vi "get_image_type.vi"(8 "error in (no error)":errorcluster, 11 "Image.lvclass in":refnum<class "Image.lvclass">) -> (0 "error out":errorcluster, 2 "Image Type":T1 items=["Grayscale (U8)", "Grayscale (I16)", "Grayscale (SGL)", "Complex (CSG)", "RGB (U32)", "HSL (U32)", "RGB (U64)", "Grayscale (U16)"], 3 "Image.lvclass out":refnum<class "Image.lvclass">, 4 "bytes per pixel":i32)   [LabVIEW 2010, in "Image.lvclass"]
uses:
  Image.lvclass
  Image.lvclass/Image.ctl
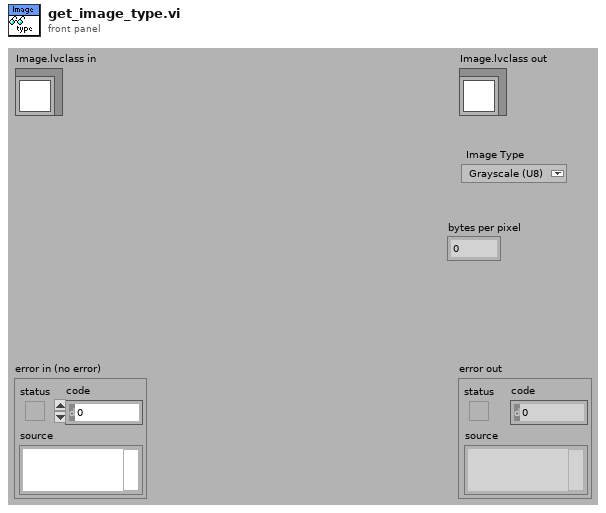
[diagram p1: front panel]
types:
  T1 = typedef "Image Type" = u32
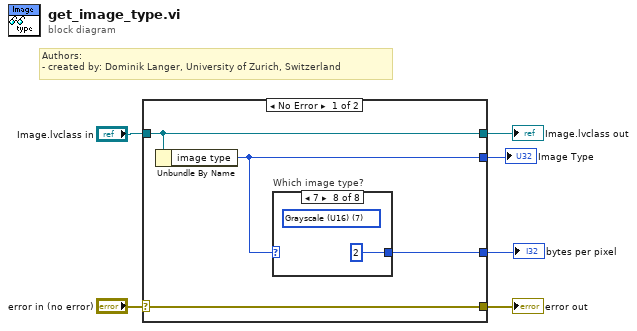
[diagram p0: block diagram]
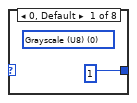
[diagram p2: hidden frame]
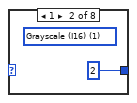
[diagram p3: hidden frame]
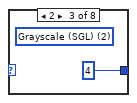
[diagram p4: hidden frame]
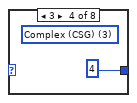
[diagram p5: hidden frame]
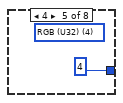
[diagram p6: hidden frame]
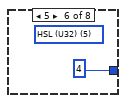
[diagram p7: hidden frame]
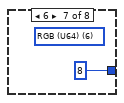
[diagram p8: hidden frame]
diagram:
  # "Authors: \n- created by: Dominik Langer, University of Zurich, Switzerland"
  n1 = case shown="No Error" "error in (no error)" {
    selector: "error in (no error)" -> [w10 w19]
    tunnel: [w10 w19] -> w5
    tunnel: [w9 w20] -> w3
    tunnel: "Image.lvclass in" -> [w9 w20]
    tunnel: [w8 _] -> w1
    tunnel: [w7 _] -> w2
    frame No Error {
      n2 = Unbundle By Name(w9) -> ("image type"=w8:T1)
      n3 = case "Which image type?" shown="7" w8 {
        tunnel: [1 2 4 4 4 4 8 2] -> w7
        frame 0, Default {
          (unwired) T1 0 items=["Grayscale (U8)", "Grayscale (I16)", "Grayscale (SGL)", "Complex (CSG)", "RGB (U32)", "HSL (U32)", "RGB (U64)", "Grayscale (U16)"] ("Image Type")
        }
        frame 1 {
          (unwired) T1 1 items=["Grayscale (U8)", "Grayscale (I16)", "Grayscale (SGL)", "Complex (CSG)", "RGB (U32)", "HSL (U32)", "RGB (U64)", "Grayscale (U16)"] ("Image Type")
        }
        frame 2 {
          (unwired) T1 2 items=["Grayscale (U8)", "Grayscale (I16)", "Grayscale (SGL)", "Complex (CSG)", "RGB (U32)", "HSL (U32)", "RGB (U64)", "Grayscale (U16)"] ("Image Type")
        }
        frame 3 {
          (unwired) T1 3 items=["Grayscale (U8)", "Grayscale (I16)", "Grayscale (SGL)", "Complex (CSG)", "RGB (U32)", "HSL (U32)", "RGB (U64)", "Grayscale (U16)"] ("Image Type")
        }
        frame 4 {
          (unwired) T1 4 items=["Grayscale (U8)", "Grayscale (I16)", "Grayscale (SGL)", "Complex (CSG)", "RGB (U32)", "HSL (U32)", "RGB (U64)", "Grayscale (U16)"] ("Image Type")
        }
        frame 5 {
          (unwired) T1 5 items=["Grayscale (U8)", "Grayscale (I16)", "Grayscale (SGL)", "Complex (CSG)", "RGB (U32)", "HSL (U32)", "RGB (U64)", "Grayscale (U16)"] ("Image Type")
        }
        frame 6 {
          (unwired) T1 6 items=["Grayscale (U8)", "Grayscale (I16)", "Grayscale (SGL)", "Complex (CSG)", "RGB (U32)", "HSL (U32)", "RGB (U64)", "Grayscale (U16)"] ("Image Type")
        }
        frame 7 {
          (unwired) T1 7 items=["Grayscale (U8)", "Grayscale (I16)", "Grayscale (SGL)", "Complex (CSG)", "RGB (U32)", "HSL (U32)", "RGB (U64)", "Grayscale (U16)"] ("Image Type")
        }
      }
    }
    frame Error {
    }
  }
  "error out" <- w5
  "Image.lvclass out" <- w3
  "bytes per pixel" <- w2
  "Image Type" <- w1
